vi "BH1750commands.vi"(6 "set res level(31-254)":u8=1, 7 "I2C Channel":u8, 8 "Error In":errorcluster, 9 "Command":u16(ring) items=["power down", "Power on", "Reset", "Continuously H- res", "Continuously H- res mode 2", "Continuously L- res", "One time H- res ", "One time H- res mode 2", "One time L res ", "Change Measurement time High bit", "Change Measurement time  Low Bit"], 10 "I2C Slave Address (0)":u8, 11 "LINX Resource":T1={"IO"=enum."Remote", "Interface"=enum."TCP", "LINX Device Config"={"Interface"=enum."TCP", "COM Port"="N/A", "TCP Configuration"={"IP Address"="panicattack", "Port"=6999}, "Device Family"=4, "Device ID"=1, "Device Name"="Raspberry Pi Model B", "TCP Ref"=refnum, "Channels"={"DI"=[2, 3, 4, 7, 8, 9, 10, 11, 14, 15, 17, 18, 22, 23, 24, 25, 27], "DO"=[2, 3, 4, 7, 8, 9, 10, 11, 14, 15, 17, 18, 22, 23, 24, 25, 27], "AI"=[], "AO"=[], "PWM"=[], "QE"=[], "UART"=[0], "I2C 2"=[0, 1], "SPI"=[0], "CAN"=[], "Servo"=[], "AI Ref (V)"=0.0, "AI Resolution (Bits)"=0, "AO Ref (V)"=0.0, "AO Resolution (Bits)"=0}}}) -> (0 "Error Out":errorcluster, 1 "Resoultion (lux)":dbl, 3 "LINX Resource out":T1={"IO"=enum."Remote", "Interface"=enum."TCP", "LINX Device Config"={"Interface"=enum."TCP", "COM Port"="N/A", "TCP Configuration"={"IP Address"="panicattack", "Port"=6999}, "Device Family"=4, "Device ID"=1, "Device Name"="Raspberry Pi Model B", "TCP Ref"=refnum, "Channels"={"DI"=[2, 3, 4, 7, 8, 9, 10, 11, 14, 15, 17, 18, 22, 23, 24, 25, 27], "DO"=[2, 3, 4, 7, 8, 9, 10, 11, 14, 15, 17, 18, 22, 23, 24, 25, 27], "AI"=[], "AO"=[], "PWM"=[], "QE"=[], "UART"=[0], "I2C 2"=[0, 1], "SPI"=[0], "CAN"=[], "Servo"=[], "AI Ref (V)"=0.0, "AI Resolution (Bits)"=0, "AO Ref (V)"=0.0, "AO Resolution (Bits)"=0}}})   [LabVIEW 2022 SP3]
uses:
  <vilib>/MakerHub/LINX/Private/Type Defs/LINX Ref.ctl
  <vilib>/MakerHub/LINX/Private/Type Defs/Platform.ctl
  <vilib>/MakerHub/LINX/Private/Type Defs/Interface.ctl
  <vilib>/MakerHub/LINX/Private/Device/Type Defs/LINX Device Config.ctl
  <vilib>/MakerHub/LINX/Private/Device/Type Defs/TCP Config.ctl
  <vilib>/MakerHub/LINX/Private/Device/Type Defs/Channels.ctl
  <vilib>/MakerHub/LINX/Private/Local IO/LinxI2cWrite.vi
  <vilib>/MakerHub/LINX/Public/Utilities/Check Channel.vi
  <vilib>/MakerHub/LINX/Private/Utilties/Generate Error.vi
  <vilib>/MakerHub/LINX/LMH-LINX.lvlib
  <vilib>/MakerHub/LINX/Private/Device/Device.lvlib
panel:
  out "String":string
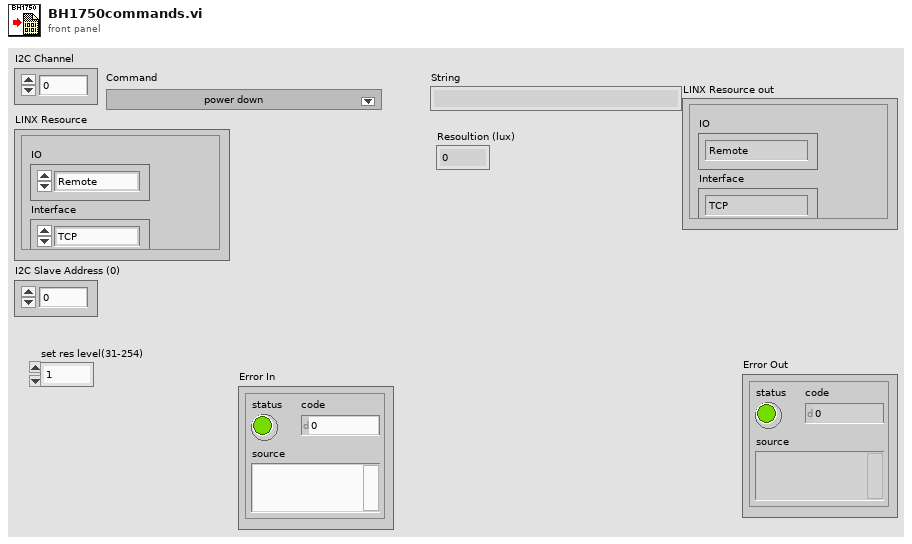
[diagram p1: front panel]
types:
  T1 = typedef "LMH-LINX.lvlib/LINX Ref.ctl" = cluster{"IO":T2, "Interface":T3, "LINX Device Config":T4}
  T2 = typedef "LMH-LINX.lvlib/Platform.ctl" = enum16{"Remote", "Local"}
  T3 = typedef "LMH-LINX.lvlib/Interface.ctl" = enum16{"Serial", "TCP"}
  T4 = typedef "LMH-LINX.lvlib/Device.lvlib/LINX Device Config.ctl" = cluster{"Interface":T3, "COM Port":refnum<visa-resource-name>, "TCP Configuration":T5, "Device Family":u8, "Device ID":u8, "Device Name":string, "TCP Ref":refnum<k5>, "Channels":T6}
  T5 = typedef "LMH-LINX.lvlib/Device.lvlib/TCP Config.ctl" = cluster{"IP Address":string, "Port":u16}
  T6 = typedef "LMH-LINX.lvlib/Channels.ctl" = cluster{"DI":u8[], "DO":u8[], "AI":u8[], "AO":u8[], "PWM":u8[], "QE":u8[], "UART":u8[], "I2C 2":u8[], "SPI":u8[], "CAN":u8[], "Servo":u8[], "AI Ref (V)":dbl, "AI Resolution (Bits)":u8, "AO Ref (V)":dbl, "AO Resolution (Bits)":u8}
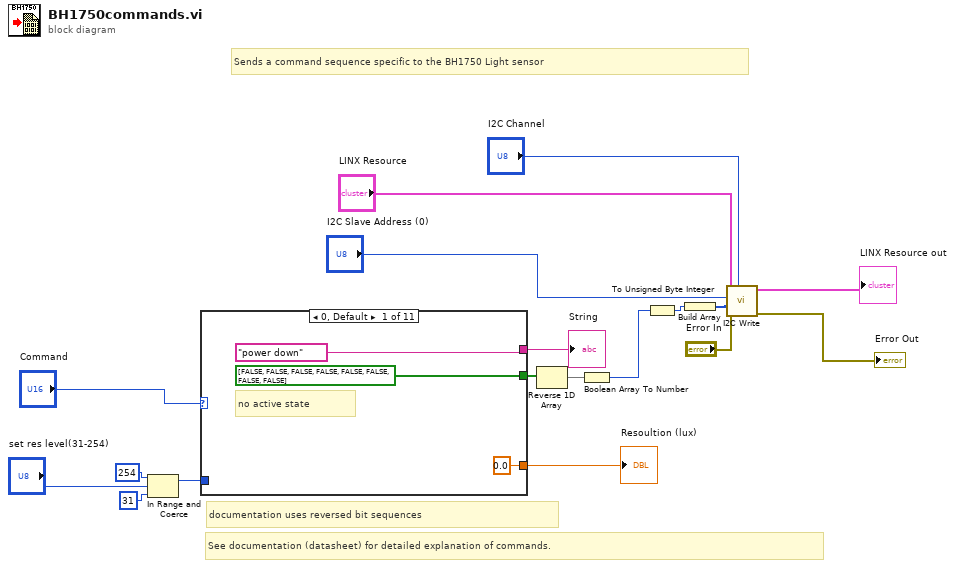
[diagram p0: block diagram]
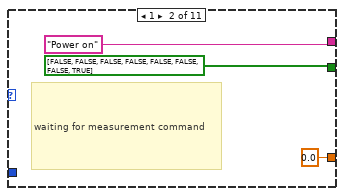
[diagram p2: hidden frame]
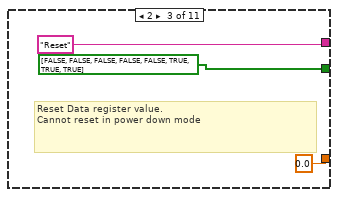
[diagram p3: hidden frame]
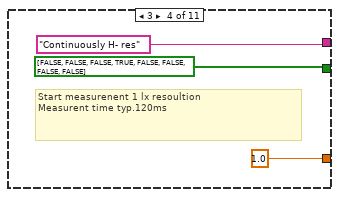
[diagram p4: hidden frame]
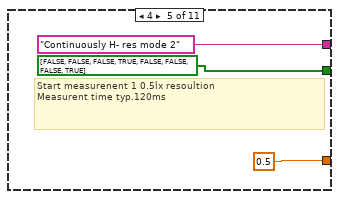
[diagram p5: hidden frame]
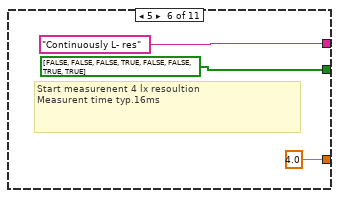
[diagram p6: hidden frame]
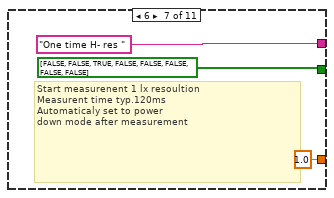
[diagram p7: hidden frame]
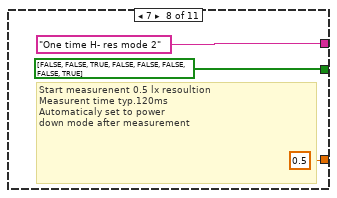
[diagram p8: hidden frame]
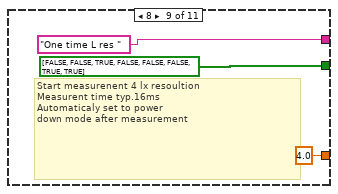
[diagram p9: hidden frame]
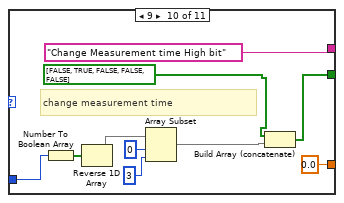
[diagram p10: hidden frame]
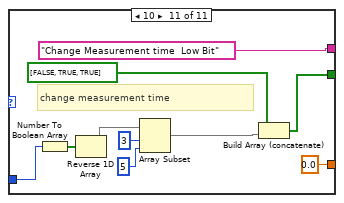
[diagram p11: hidden frame]
diagram:
  # "See documentation (datasheet) for detailed explanation of commands."
  # "Sends a command sequence specific to the BH1750 Light sensor"
  # "documentation uses reversed bit sequences"
  n1 = In Range and Coerce(upper limit=254 ("lower limit"), x="set res level(31-254)", lower limit=31) -> (coerced(x)=w11:i32)  [unwired: 1 out]
  n2 = case shown="0, Default" "Command" {
    tunnel: ["power down" "Power on" "Reset" "Continuously H- res" "Continuously H- res mode 2" "Continuously L- res" "One time H- res " "One time H- res mode 2" "One time L res " "Change Measurement time High bit" "Change Measurement time  Low Bit"] -> w17
    tunnel: [bool[] [FALSE, FALSE, FALSE, FALSE, FALSE, FALSE, FALSE, FALSE] ("Boolean array") bool[] [FALSE, FALSE, FALSE, FALSE, FALSE, FALSE, FALSE, TRUE] ("Boolean array") bool[] [FALSE, FALSE, FALSE, FALSE, FALSE, TRUE, TRUE, TRUE] ("Boolean array") bool[] [FALSE, FALSE, FALSE, TRUE, FALSE, FALSE, FALSE, FALSE] ("Boolean array") bool[] [FALSE, FALSE, FALSE, TRUE, FALSE, FALSE, FALSE, TRUE] ("Boolean array") bool[] [FALSE, FALSE, FALSE, TRUE, FALSE, FALSE, TRUE, TRUE] ("Boolean array") bool[] [FALSE, FALSE, TRUE, FALSE, FALSE, FALSE, FALSE, FALSE] ("Boolean array") bool[] [FALSE, FALSE, TRUE, FALSE, FALSE, FALSE, FALSE, TRUE] ("Boolean array") bool[] [FALSE, FALSE, TRUE, FALSE, FALSE, FALSE, TRUE, TRUE] ("Boolean array") w49 w58] -> w13
    tunnel: w11 -> [_ _ _ _ _ _ _ _ _ w53 w60]
    tunnel: [0.0 0.0 0.0 1.0 0.5 4.0 1.0 0.5 4.0 0.0 0.0] -> w1
    frame 0, Default {
      # "no active state"
    }
    frame 1 {
      # "waiting for measurement command"
    }
    frame 2 {
      # "Reset Data register value.\nCannot reset in power down mode"
    }
    frame 3 {
      # "Start measurenent 1 lx resoultion\nMeasurent time typ.120ms"
    }
    frame 4 {
      # "Start measurenent 1 0.5lx resoultion\nMeasurent time typ.120ms"
    }
    frame 5 {
      # "Start measurenent 4 lx resoultion\nMeasurent time typ.16ms"
    }
    frame 6 {
      # "Start measurenent 1 lx resoultion\nMeasurent time typ.120ms\nAutomaticaly set to power \ndown mode after measurement"
    }
    frame 7 {
      # "Start measurenent 0.5 lx resoultion\nMeasurent time typ.120ms\nAutomaticaly set to power \ndown mode after measurement"
    }
    frame 8 {
      # "Start measurenent 4 lx resoultion\nMeasurent time typ.16ms\nAutomaticaly set to power \ndown mode after measurement"
    }
    frame 9 {
      # "change measurement time"
      n3 = Number To Boolean Array(number=w53) -> (Boolean array=w54:bool[])
      n4 = Reverse 1D Array(array=w54) -> (reversed array=w52:bool[])
      n5 = Array Subset(array=w52, index=0, length=3) -> (w51:bool[])
      n6 = Build Array (concatenate)(bool[] [FALSE, TRUE, FALSE, FALSE, FALSE] ("Boolean array"), w51) -> (w49:bool[])
    }
    frame 10 {
      # "change measurement time"
      n7 = Number To Boolean Array(number=w60) -> (Boolean array=w64:bool[])
      n8 = Reverse 1D Array(array=w64) -> (reversed array=w63:bool[])
      n9 = Array Subset(array=w63, index=3, length=5) -> (w62:bool[])
      n10 = Build Array (concatenate)(bool[] [FALSE, TRUE, TRUE] ("Boolean array"), w62) -> (w58:bool[])
    }
  }
  "String" <- w17
  "Resoultion (lux)" <- w1
  n11 = Reverse 1D Array(array=w13) -> (reversed array=w12:bool[])
  n12 = Boolean Array To Number(Boolean array=w12) -> (number=w8:u32)
  n13 = To Unsigned Byte Integer(number=w8) -> (unsigned 8bit integer=w7:u8)
  n14 = Build Array(w7) -> (w6:u8[])
  n15 = call <vilib>:"I2C Write.vi"("I2C Channel"="I2C Channel", "Error In"="Error In", "Data"=w6, "I2C Slave Address (0)"="I2C Slave Address (0)", "LINX Resource"="LINX Resource") -> ("Error Out"=→"Error Out":errorcluster, "LINX Resource"=→"LINX Resource out":T1)  [unwired: 5 in]
